vi "ARN Test Konfig v2.vi"() -> ()   [LabVIEW 2020, in "EPA 1065.lvlib" / "ARN Test 1065-305.lvlib"]
uses:
  ARN Test 1065-305.lvlib
  Visualisierungs Elemente/Zahlen-Ausgabefeld.ctl
  Allgemeine Einstellungen.ctl
  Seiten/System Einstellungen V2/Analysatoren.ctl
  T90 1065-308/Modus.ctl
  Seiten/System Einstellungen V2/Gasflasche Auswahl.ctl
  Seiten/System Einstellungen V2/Konfig Gasflasche.ctl
  T90 1065-308/Ergebnis.ctl
  Aktion FGV ARN Daten.ctl
  Seiten/FT-IR/FGV FT-IR Gasliste Aktionen.ctl
  Aktion FGV ARN Test.ctl
  Sprachverwaltung/FGV Aktion Tabelle zerlegen.ctl
  Aktion FGV Graphen Daten.ctl
  Seiten/System Einstellungen V2/Aktion FGV Gasbottledefinition.ctl
  PDF_Interface/PDF Interface Helper/PDFResultPictures.ctl
  Aktion FGV ARN Protokoll.ctl
  Messdaten/Aktionen FGV Messdaten.ctl
  Allgemeine VIs/Aktion Wertaenderung Gasliste.ctl
  Aktion FGV Protokoll.ctl
  Seiten/Gaszuordnung AO/FGV Gaszuordnung Grenzen&Einheit Aktion.ctl
  Allgemeine VIs/Aktion Test Status.ctl
  Funktionstasten/Funktionstasten-Aktion.ctl
  Funktionstasten/Zustaende.ctl
  Seiten/FT-IR/FGV FT-IR Parameter.vi
  Allgemein/allgemeine Sub-VIs.lvlib
  Seiten/FT-IR/FT-IR.lvlib
  Messdaten/Messdaten.lvlib
  Seiten/Grafik/Grafik.lvlib
  Funktionstasten/Funktionstasten.lvlib
  Seiten/Gaszuordnung AO/Gaszuordnung AO.lvlib
  EPA 1065.lvlib
  Sprachverwaltung/Sprachverwaltung.lvlib
  Seiten/System Einstellungen V2/System Einstellungen V2.lvlib
  PDF_Interface/PDF Interface Helper/PDF Interface Helper.lvlib
  T90 1065-308/T90 Test 1065-308.lvlib
panel:
  out "ARN Result PDF":waveform(sgl)(graph) caption="T90"
  out "Ergebnis PDF FALSE":T1 caption="Ergebnis 2"
  out "Ergebnis PDF TRUE":T1 caption="Ergebnis 1"
  in  "Systemeinstellung":bool caption="Gasliste geändert"
  in  "Gasliste geändert":bool
  in  "Registerkarte":enum32{"Settings", "ARN Test", "Result"}(tab)
  in  "ARN Konfig Daten":T2={"Bearbeiter:"="", "Analysator"="FT-IR", "Komponente:"=0, "Gasflaschen Nr.:"="", "Accuracy"=0.0, "Sollwert"=0.0, "Modus"=0, "Pfad:"=path "D:/IAG_Data/Log", "Textname:"="", "CG Aufschaltzeit:"=120.0, "Einheit"="", "N2 Aufschaltzeit:"=120.0, "Gasflasche"=0, "Konfig Gasflasche"=FALSE} {"Gasflasche" items=["----"=10000, "IAG O2"=0, "IAG C2H2"=1, "IAG C2H4"=2, "IAG NH3 200"=3, "IAG NH3 2000"=4, "IAG NH3 3000"=5, "IAG CO 5%"=6, "IAG Propane 2%"=7, "IAG NO 1000"=8, "IAG SO2"=9, "IAG C3H6"=10, "IAG CO2"=11, "IAG CO"=12, "IAG N2O"=13, "IAG N2O 100"=14, "IAG NO2 1000"=15, "IAG NO2 100"=16, "IAG CH4"=17, "IAG Propane"=18, "IAG NO 5000"=19, "Hansi"=20, "IAG MG"=21]; "Komponente:" items=["N2O (300) LP 191C (1of2)"=3, "N2O (1000) LP 191C (2of2)"=29, "N2O autorange (1000)"=40]; "Modus" items=["CG zu PNS", "CG zu Entnahmestelle"]; "N2 Aufschaltzeit:" min=10.0; "CG Aufschaltzeit:" min=10.0}
  in  "Speichern":bool
  out "Einheit":string
  out "Komponente":string caption="Komponente:"
  out "Status":string
  out "ARN":waveform(sgl)(graph) caption="T90"
  in  "Test Start":bool
  in  "Abbrechen":bool
  out "Istwert":T7 caption="Istwert:" format="%.2f"
  out "Mwert":sgl format="%.3f"
  out "PMwert":sgl format="%.3f"
  in  "Textfile":bool caption="Abbrechen"
  out "Einheit Noise 2":string
  out "Einheit Wiederh. 2":string
  out "Einheit Genauigkeit 2":string
  out "Einheit Noise":string
  out "Einheit Wiederh.":string
  out "Ergebnis 3":T1
  out "Ergebnis 2":T1
  out "Ergebnis 1":T1
  out "Rauschen":string
  out "Rauschen Grenze":string caption="Rauschen:"
  out "Wiederholgenauigkeit":string
  out "Genauigkeit":string
  out "Wiederholgenauigkeit Grenze":string caption="Wiederholgenauigkeit:"
  out "Genauigkeit Grenze":string caption="Genauigkeit:"
  out "Einheit Genauigkeit":string
  out "ARN Result":waveform(sgl)(graph) caption="T90"
  in  "Print PDF":bool caption="Abbrechen"
  out "Tabelle":string[][](table)
  out "Komponente 2":string caption="Komponente:"
  # "ANR Test EPA §1065.305"
  # "Allgemeine Einstellungen"
  # "Protokoll Einstellung"
  # "%"
  # "sec."
  # "sec."
  # "±"
  # "x"
  # "Grenzen"
  # "Ergebnis"
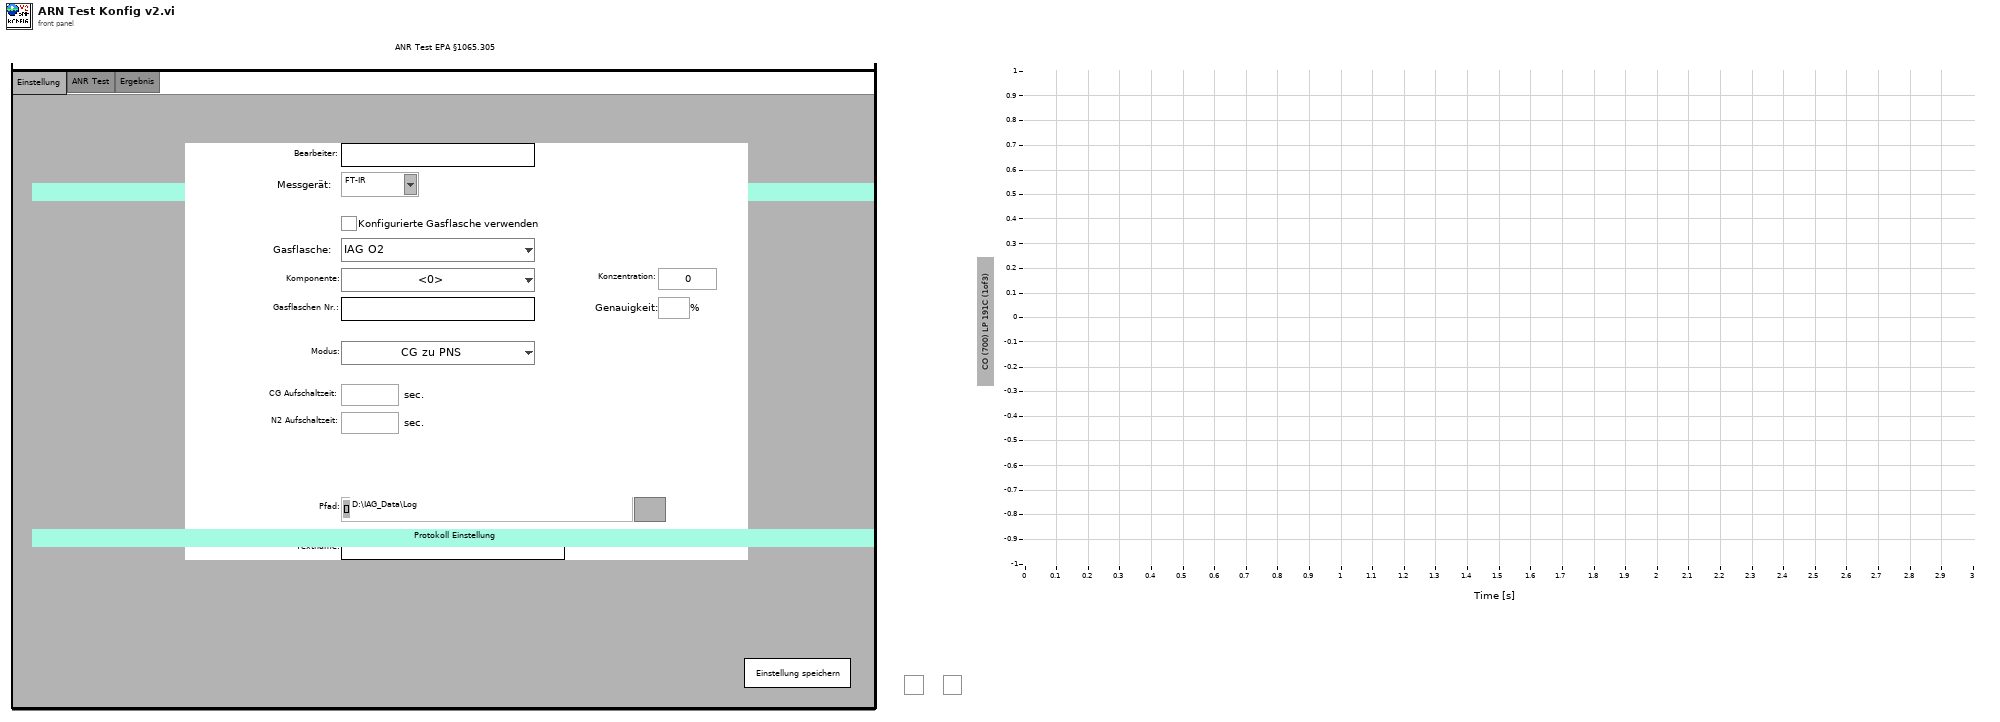
[diagram p1: front panel]
types:
  T1 = typedef "EPA 1065.lvlib/T90 Test 1065-308.lvlib/Ergebnis.ctl" = bool
  T2 = typedef "EPA 1065.lvlib/ARN Test 1065-305.lvlib/Allgemeine Einstellungen.ctl" = cluster{"Bearbeiter:":string, "Analysator":T3, "Komponente:":u16, "Gasflaschen Nr.:":string, "Accuracy":dbl, "Sollwert":dbl, "Modus":T4, "Pfad:":path, "Textname:":string, "CG Aufschaltzeit:":dbl, "Einheit":string, "N2 Aufschaltzeit:":dbl, "Gasflasche":T5, "Konfig Gasflasche":T6}
  T3 = typedef "System Einstellungen V2.lvlib/Analysatoren.ctl" = string
  T4 = typedef "EPA 1065.lvlib/T90 Test 1065-308.lvlib/Modus.ctl" = u16
  T5 = typedef "System Einstellungen V2.lvlib/Gasflasche Auswahl.ctl" = u16
  T6 = typedef "System Einstellungen V2.lvlib/Konfig Gasflasche.ctl" = bool
  T7 = typedef "Zahlen-Ausgabefeld.ctl" = sgl
  T8 = typedef "System Einstellungen V2.lvlib/Aktion FGV Gasbottledefinition.ctl" = enum16{"lesen", "schreiben", "löschen", "laden", "speichern", "exportieren", "importieren"}
  T9 = typedef "EPA 1065.lvlib/ARN Test 1065-305.lvlib/Aktion FGV ARN Daten.ctl" = enum16{"Lesen", "laden", "speichern", "ARN Daten", "Rohdaten", "Rohdaten löschen", "Zeitstempel", "SNR Ergebnis"}
  T10 = typedef "EPA 1065.lvlib/ARN Test 1065-305.lvlib/Aktion FGV Graphen Daten.ctl" = enum16{"init", "lesen", "Daten schreiben"}
  T11 = typedef "Sprachverwaltung.lvlib/FGV Aktion Tabelle zerlegen.ctl" = enum16{"laden", "vereinzeln", "speichern"}
  T12 = enum16{"init", "lesen", "ARN Test aktiv", "ARN Test inaktiv"}
  T13 = typedef "EPA 1065.lvlib/ARN Test 1065-305.lvlib/Aktion FGV ARN Test.ctl" = enum16{"leerlauf", "init", "lesen", "CG aufschalten", "Aufschaltzeit abwarten", "aufzeichnen vorbereiten", "aufzeichnen", "berechnen", "auswerten", "fertig", "0-Gas aufschalten", "0-Gas abwarten"}
  T14 = typedef "FT-IR.lvlib/FGV FT-IR Gasliste Aktionen.ctl" = enum16{"lesen", "Gasliste FT-IR", "Gasliste ausgelesen", "laden", "speichern", "löschen"}
  T15 = typedef "PDF Interface.lvlib/PDF Interface Helper.lvlib/PDFResultPictures.ctl" = cluster{"Yes Ctl Refnum":refnum<vi>, "No Ctl Refnum":refnum<vi>}
  T16 = typedef "String - Ausgabefeld.ctl" = string
  T17 = typedef "System Einstellungen V2.lvlib/Gasflasche gesamt.ctl" = cluster{"Gasflasche":T18, "Trägergas":T19, "Komponenten":T20[]}
  T18 = typedef "System Einstellungen V2.lvlib/Gasflasche.ctl" = cluster{"Gasname für die Auswahl":string, "Chargennummer":string, "Ablaufdatum":timestamp}
  T19 = typedef "System Einstellungen V2.lvlib/Traegergas.ctl" = string
  T20 = typedef "System Einstellungen V2.lvlib/Gasflaschenkomponente.ctl" = cluster{"Gasauswahl":string, "Konzentration IST":dbl, "Einheit":string, "Genauigkeit":dbl}
  T21 = cluster{"Komponente:":u16, "Sollwert":dbl, "Accuracy":dbl, "Einheit":string, "Gasflaschen Nr.:":string}
  T22 = typedef "EPA 1065.lvlib/Aktion Wertaenderung Gasliste.ctl" = enum16{"Init", "lesen", "Gasliste geändert", "ARN inaktiv", "LEAK inaktiv", "Interference 366 inaktiv", "T90 inaktiv", "Interference 375 inaktiv", "Chiller inaktiv", "FID O2 inaktiv", "FID Opti inaktiv", "Drift inaktiv", "Pre Test inaktiv", "LinV2 inaktiv", "HovaCAL Interference inaktiv"}
  T23 = typedef "Messdaten.lvlib/Aktionen FGV Messdaten.ctl" = enum16{"lesen", "schreiben", "löschen", "Mittelwerte", "Komponente"}
  T24 = typedef "EPA 1065.lvlib/ARN Test 1065-305.lvlib/Aktion FGV ARN Protokoll.ctl" = enum16{"lesen", "Tab. schreiben", "Protokoll ausw.", "Protokoll speichern", "Textdatei speichern"}
  T25 = typedef "EPA 1065.lvlib/ARN Test 1065-305.lvlib/Aktion FGV Protokoll.ctl" = enum16{"lesen", "schreiben", "Graph"}
  T26 = typedef "Gaszuordnung AO.lvlib/FGV Gaszuordnung Grenzen&Einheit Aktion.ctl" = enum16{"Lesen", "Schreiben Min", "Schreiben Max", "Laden", "Speichern"}
  T27 = typedef "EPA 1065.lvlib/Aktion Test Status.ctl" = enum16{"init", "lesen", "prüfen", "Interference 366", "Interference 375", "Chiller läuft", "Drift läuft", "Pre Test läuft", "FID Optimization läuft", "FID Interference läuft", "HovaCAL Interference", "LinV2"}
  T28 = typedef "Funktionstasten.lvlib/Zustaende.ctl" = enum16{"Standby", "Pause", "Eco", "Messen", "Kalibrieren", "Spülen Filter", "Spülen Leitung", "Umgebungsluft", "0-Gas", "Cal-Gas", "CG zu PNS", "-------------", "Init 1", "Init 2", "Init 3", "Init 4", "Messen vorbereiten", "Messen durchführen", "Exit"}
  T29 = typedef "Funktionstasten.lvlib/Funktionstasten-Aktion.ctl" = enum16{"Initialisieren", "Zustand setzen", "Taste gedrückt", "Fehler speichern", "Lesen", "Manuell", "Remote", "Bitparallel", "Samplepoint", "Zeit Prüfen", "reset Umschalten"}
  T30 = typedef "EPA 1065.lvlib/Aktive Tests Cluster.ctl" = cluster{"ANR läuft":bool, "T90 läuft":bool, "Leak läuft":bool, "Interference 366 läuft":bool, "Interference 375 läuft":bool, "Chiller läuft":bool, "FID Interference läuft":bool, "FID optimization läuft":bool, "Drift läuft":bool, "Pre-test läuft":bool, "HovaCAL Interference läuft":bool, "LinV2 läuft":bool}
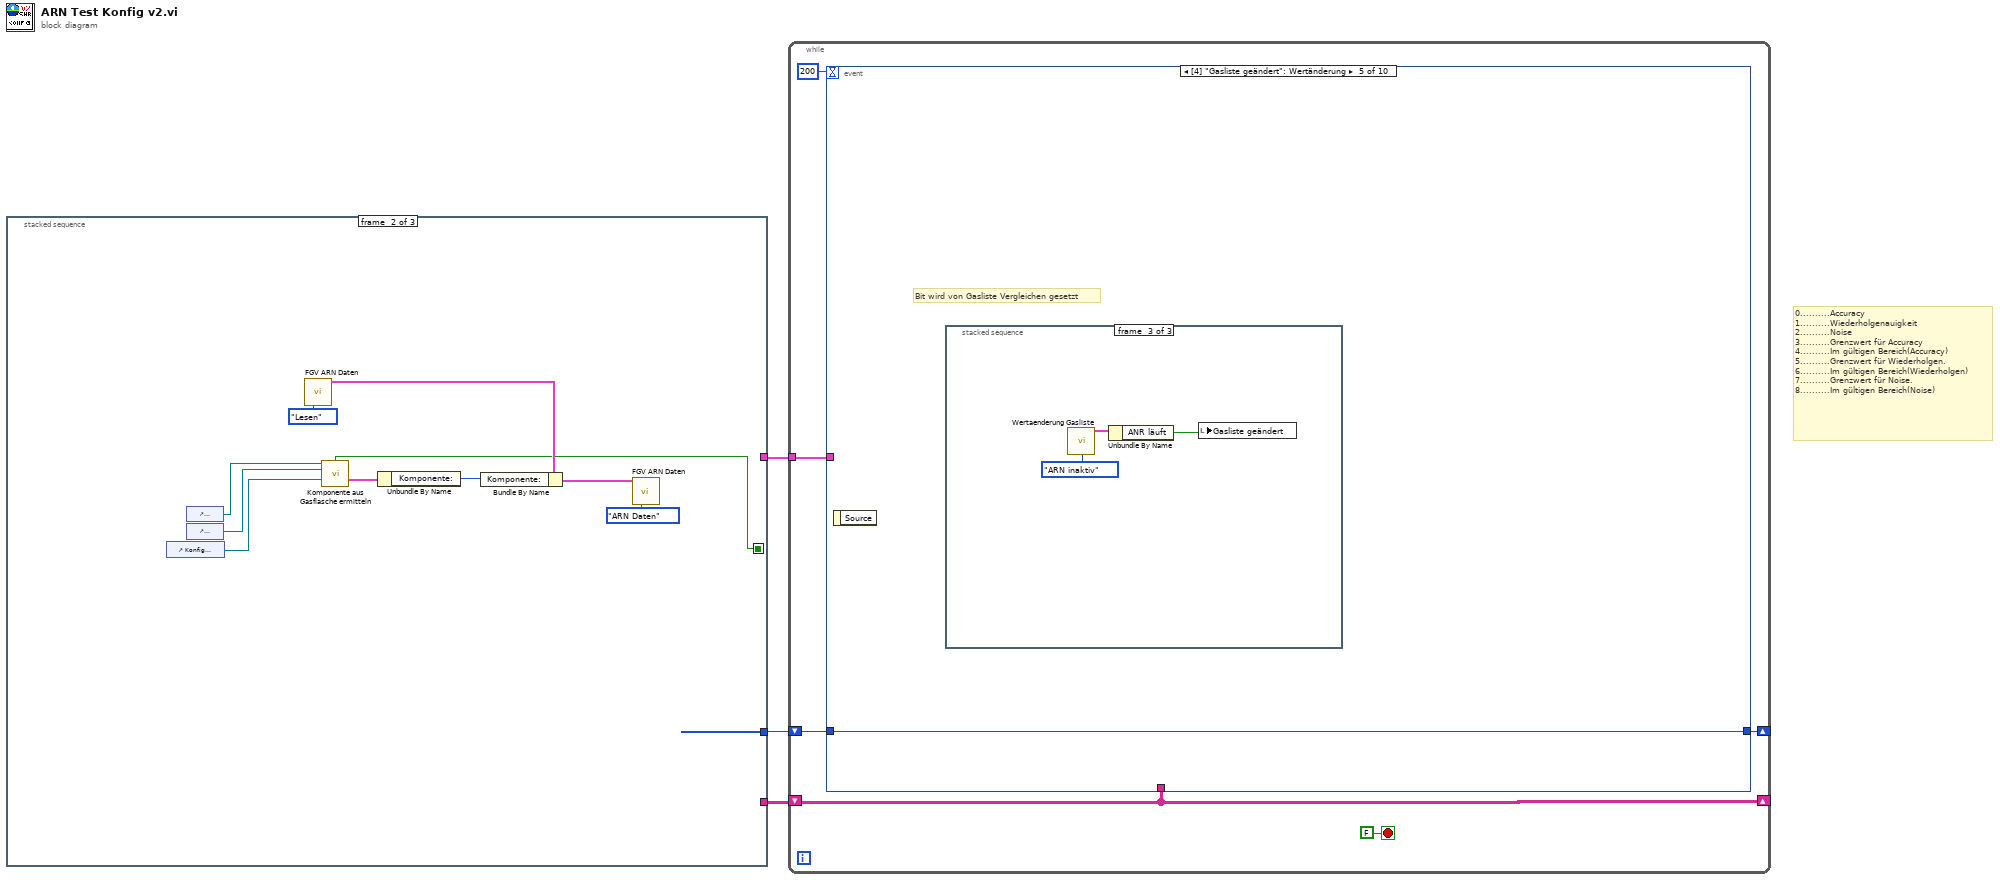
[diagram p0: block diagram]
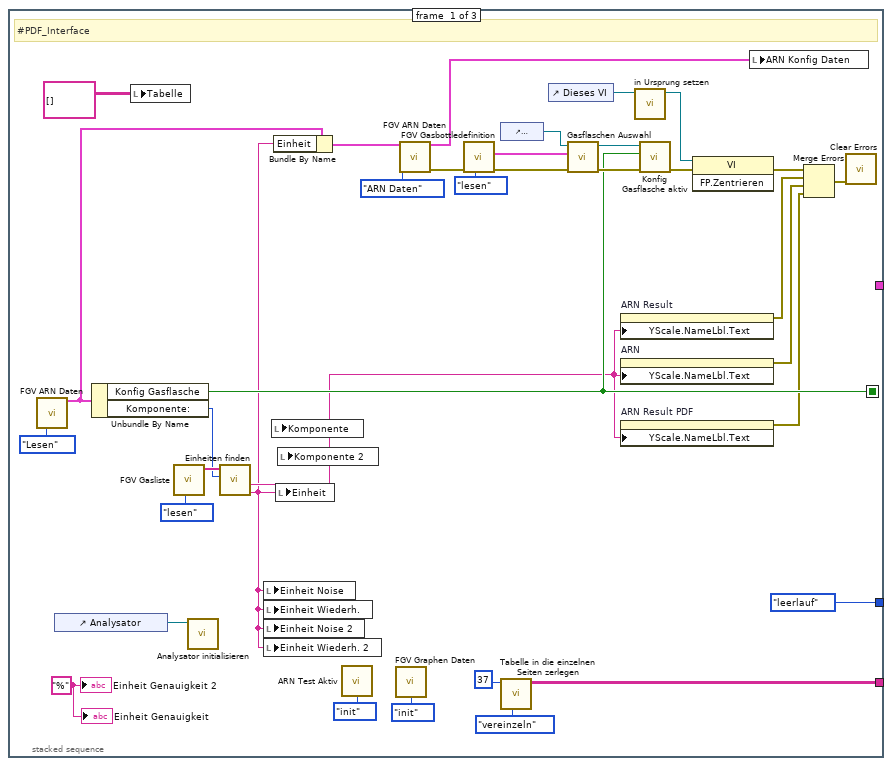
[diagram p2: hidden frame]
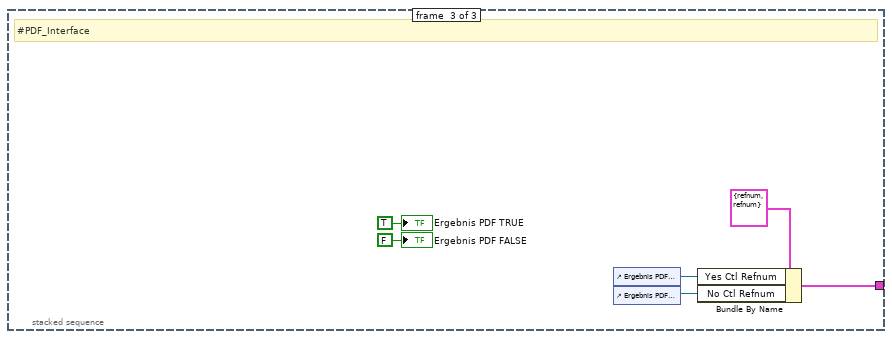
[diagram p3: hidden frame]
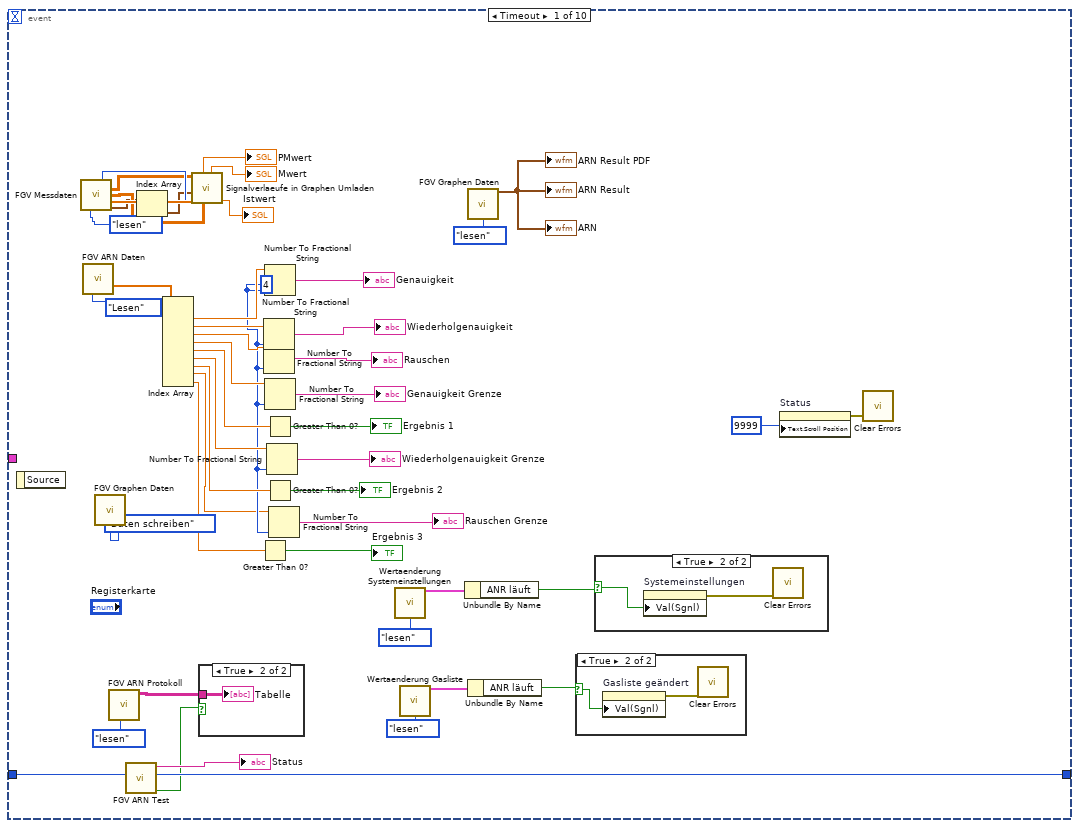
[diagram p4: hidden frame]
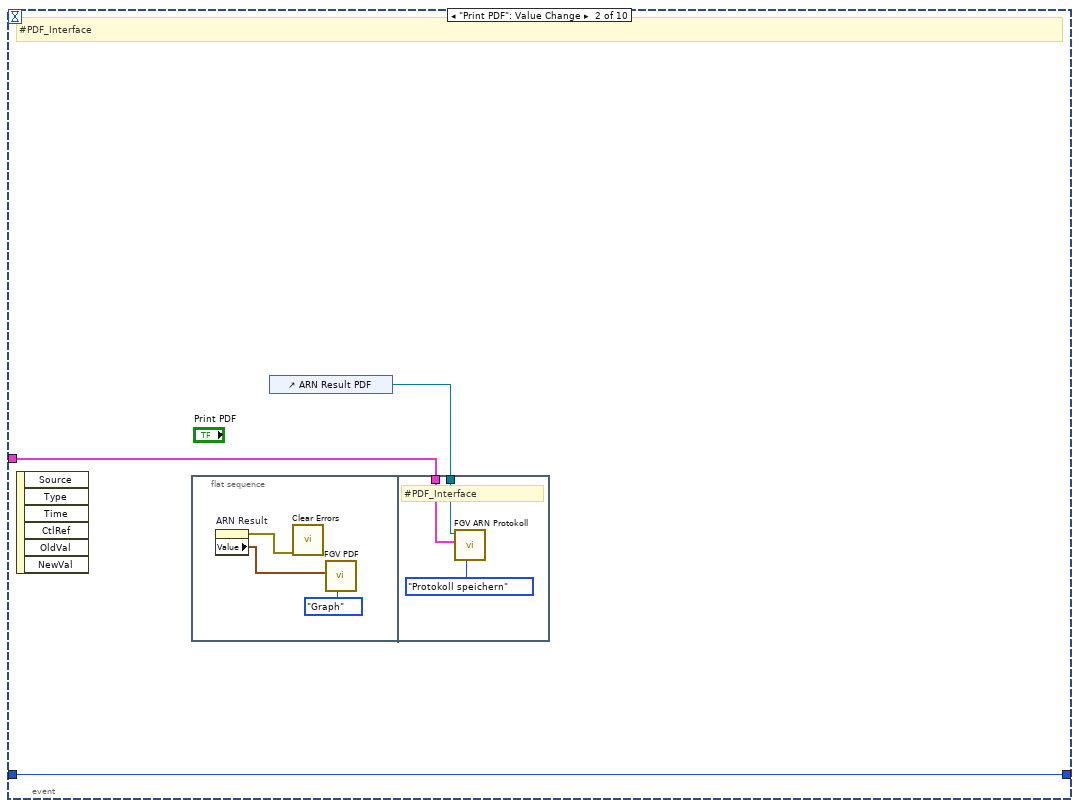
[diagram p8: hidden frame]
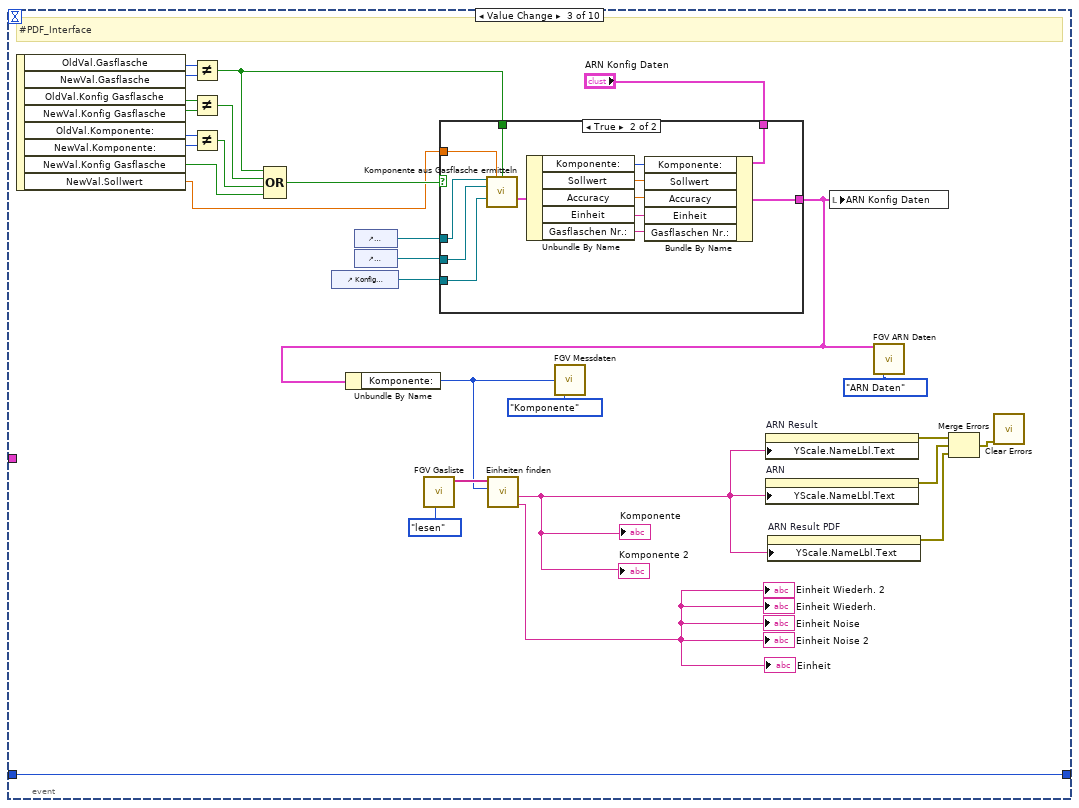
[diagram p9: hidden frame]
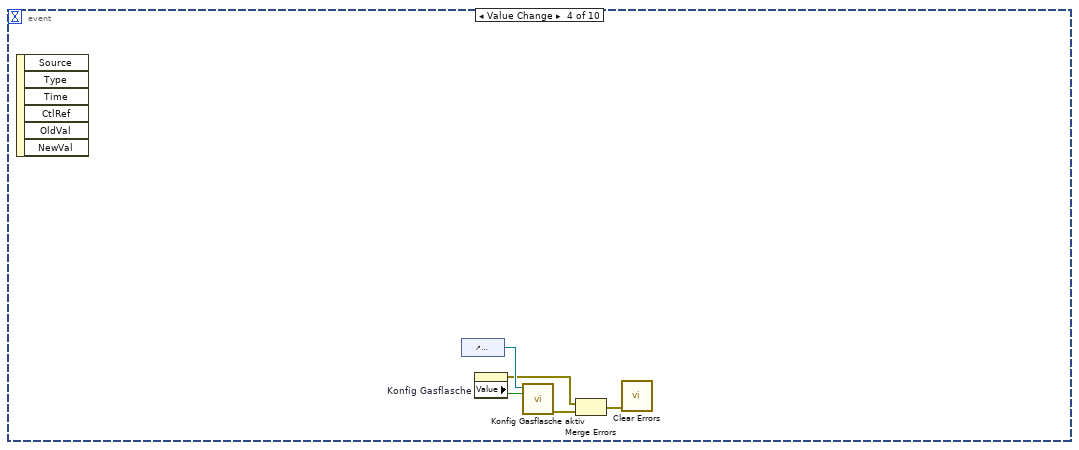
[diagram p11: hidden frame]
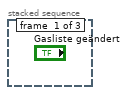
[diagram p12: hidden frame]
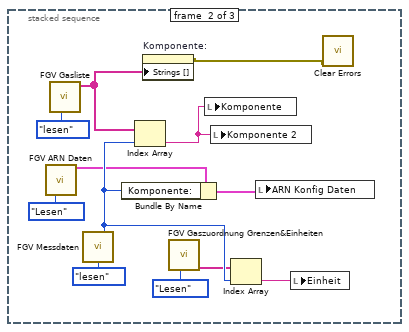
[diagram p13: hidden frame]
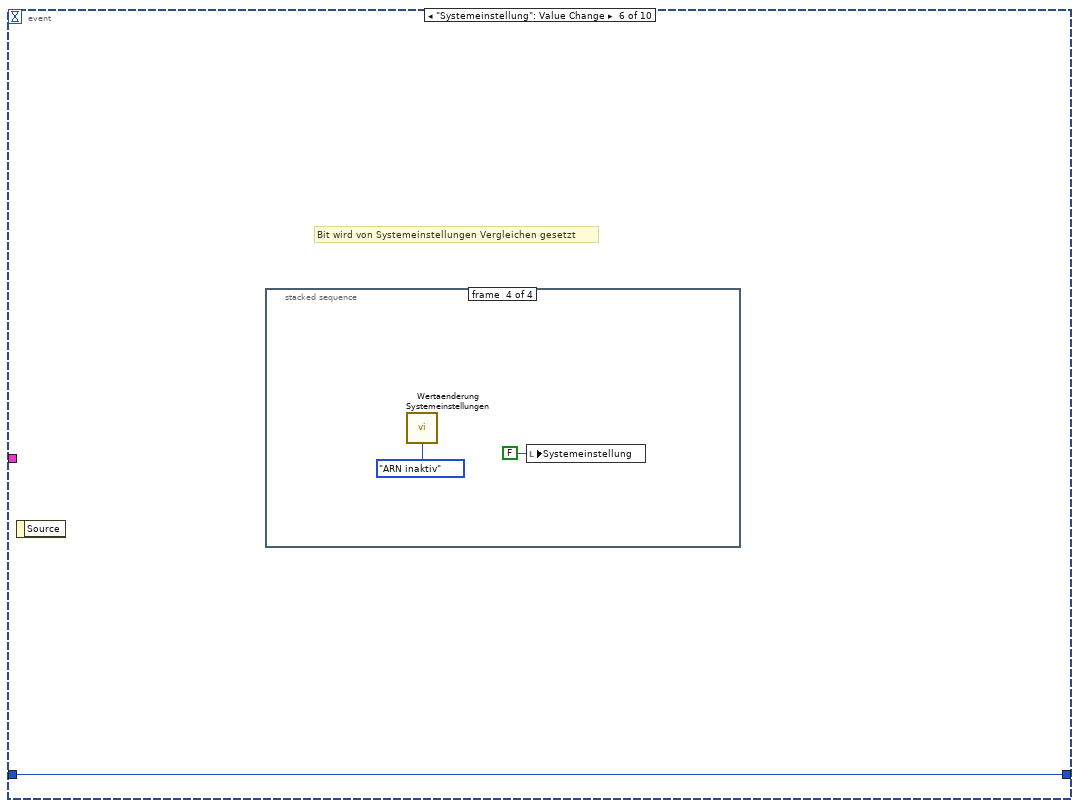
[diagram p14: hidden frame]
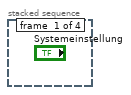
[diagram p15: hidden frame]
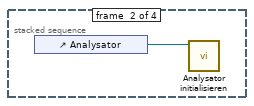
[diagram p16: hidden frame]
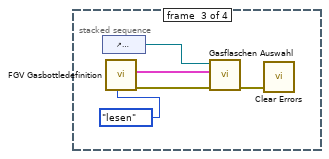
[diagram p17: hidden frame]
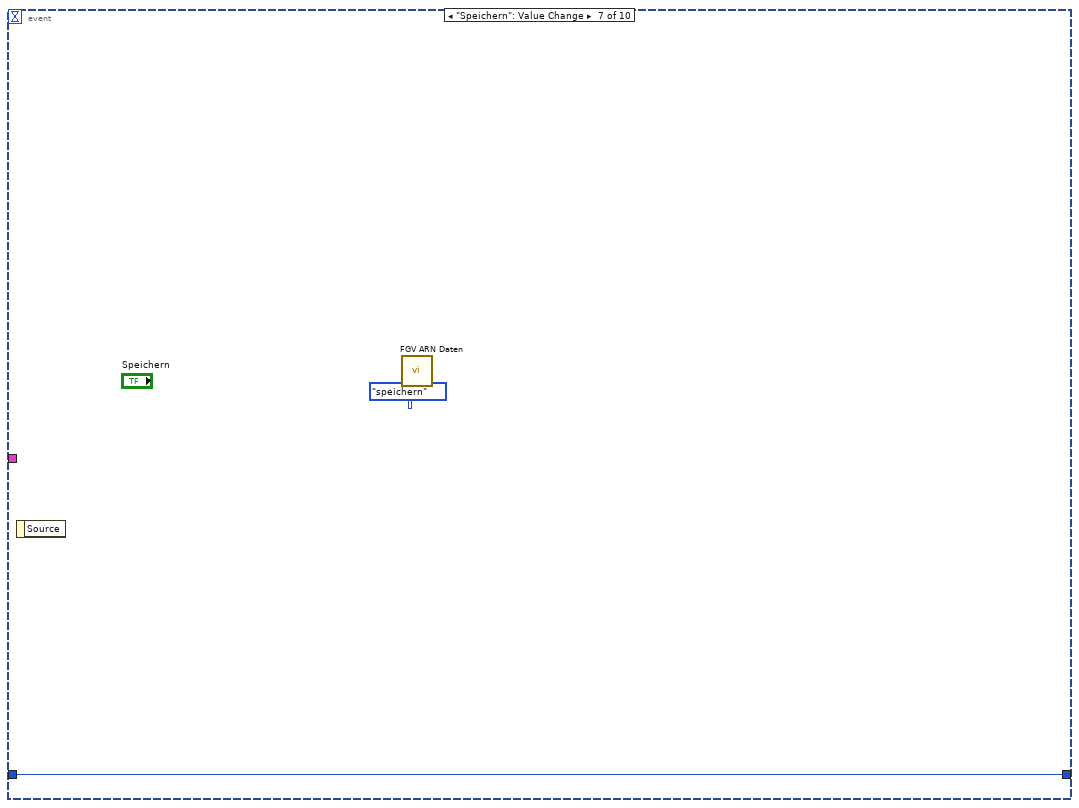
[diagram p18: hidden frame]
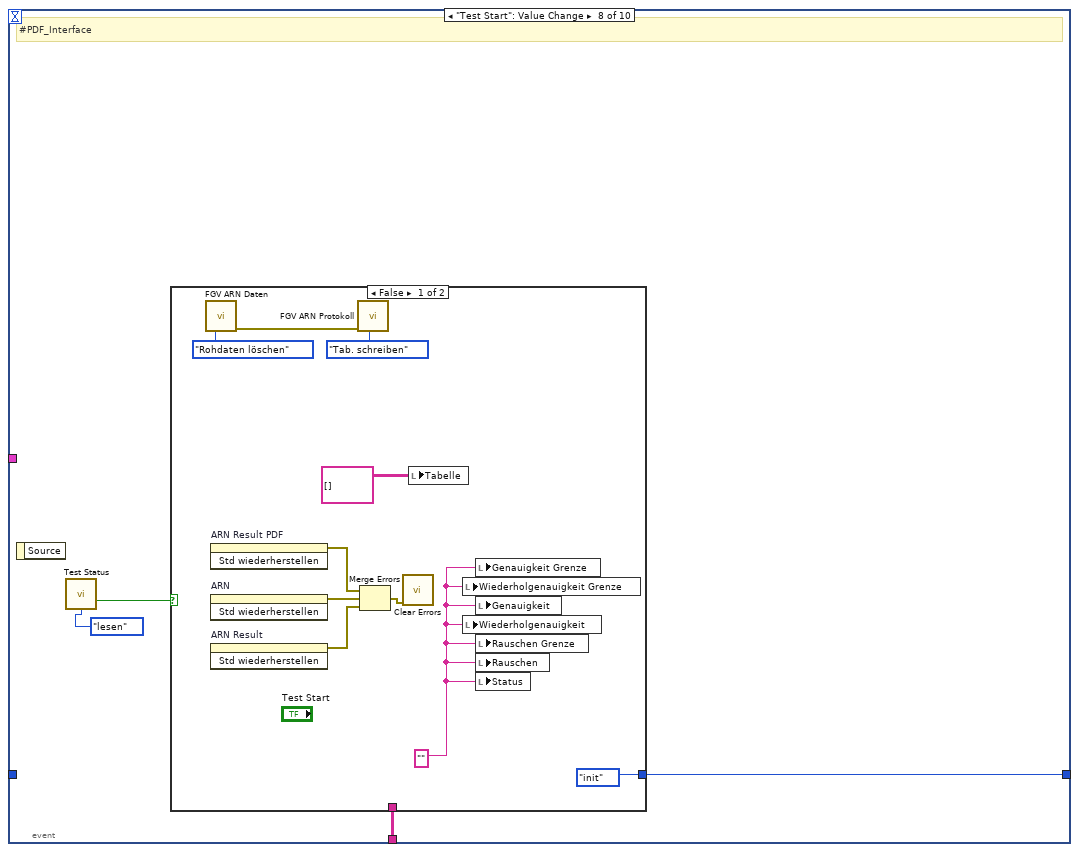
[diagram p19: hidden frame]
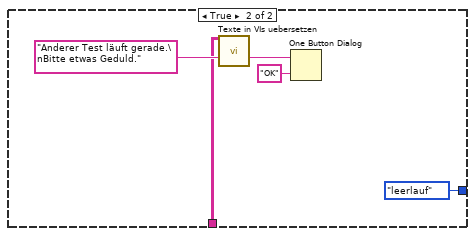
[diagram p20: hidden frame]
diagram:
  # "0..........Accuracy\n1..........Wiederholgenauigkeit\n2..........Noise\n3..........Grenzwert für Accuracy\n4..........Im gültigen Bereich(Accuracy)\n5..........Grenzwert für Wiederholgen.\n6..........Im gültigen Bereich(Wiederholgen)\n7..........Grenzwert für Noise.\n8..........Im gültigen Bereich(Noise)"
  n1 = stacked-sequence {
    seq-local: [w10 _ _] -> [_ w38 _]
    tunnel: [Aktion_FGV_ARN_Test."leerlauf" ("Aktion") _ _] -> w3
    tunnel: [w27 _ _] -> w2
    tunnel: [_ _ w48] -> w1
    frame #0 {
      w23 = "%" ("Einheit Genauigkeit 2")
      # "#PDF_Interface"
      n2 = call "FGV ARN Daten.vi"("Aktion"=Aktion_FGV_ARN_Daten."Lesen") -> ("ARN Konfig Daten"=w20:T2)  [unwired: 9 in, 5 out]
      n3 = control-ref of="Analysator"() -> (w11:refnum<vi>)
      n4 = Unbundle By Name(w20) -> ("Konfig Gasflasche"=w10:T6, "Komponente:"=w5:u16)
      n5 = local write "Tabelle"(string[][] [] ("Tabellenelement")) -> ()
      n6 = call "FGV Gasliste.vi"("Aktionen"=FGV_FT-IR_Gasliste_Aktionen."lesen") -> ("Aktuelle Gasliste FT-IR"=w8:T16[])  [unwired: 8 in, 2 out]
      n7 = call "Analysator initialisieren.vi"("Referenz Analysator"=w11) -> ()  [unwired: 9 in, 2 out]
      n8 = call "Einheiten finden.vi"("Komponente"=w5, "Aktuelle Gasliste gesamt"=w8) -> ("Einheit in String"=w6:string, "Komponenten Name"=w7:T16)  [unwired: 8 in]
      n9 = local write "Einheit Noise"(w6) -> ()
      n10 = local write "Einheit Wiederh."(w6) -> ()
      n11 = local write "Einheit Noise 2"(w6) -> ()
      n12 = local write "Einheit Wiederh. 2"(w6) -> ()
      n13 = local write "Komponente"(w7) -> ()
      n14 = Bundle By Name(cluster=w20, "Einheit"=w6) -> (w24:T2)
      n15 = local write "Einheit"(w6) -> ()
      n16 = local write "Komponente 2"(w7) -> ()
      n17 = call "ARN Test Aktiv.vi"("Aktion"=T12."init") -> ()  [unwired: 13 in, 2 out]
      n18 = call "FGV Graphen Daten.vi"("Aktion"=Aktion_FGV_Graphen_Daten."init") -> ()  [unwired: 12 in, 3 out]
      n19 = call "FGV ARN Daten.vi"("ARN Konfig Daten"=w24, "Aktion"=Aktion_FGV_ARN_Daten."ARN Daten") -> ("ARN Konfig Daten"=w14:T2, "error out"=w13:errorcluster)  [unwired: 8 in, 4 out]
      n20 = call "FGV Gasbottledefinition.vi"("Aktion"=Aktion_FGV_Gasbottledefinition."lesen", "error in (no error)"=w13) -> ("error out"=w19:errorcluster, "Gasflaschen Liste gesamt"=w18:T17[])  [unwired: 7 in, 1 out]
      n21 = control-ref of="Gasflasche"() -> (w17:refnum<vi>)
      n22 = call "Tabelle in die einzelnen Seiten zerlegen.vi"("Aktion"=FGV_Aktion_Tabelle_zerlegen."vereinzeln", "Index (Seite)"=37) -> ("Sprachliste"=w27:string[][])  [unwired: 7 in, 2 out]
      n23 = control-ref of="Dieses VI"() -> (w33:refnum<vi>)
      n24 = call "Gasflaschen Auswahl.vi"("error in (no error)"=w19, "Gasflaschen Liste gesamt"=w18, "Ring (Eingang)"=w17) -> ("error out"=w15:errorcluster)  [unwired: 8 in]
      n25 = property on="ARN Result" class="SVGraph (strikt)"("YScale.NameLbl.Text"=w7) -> (error out=w22:errorcluster)  [unwired: 2 in, 1 out]
      n26 = property on="ARN" class="SVGraph (strikt)"("YScale.NameLbl.Text"=w7) -> (error out=w21:errorcluster)  [unwired: 2 in, 1 out]
      n27 = property on="ARN Result PDF" class="SVGraph (strikt)"("YScale.NameLbl.Text"=w7) -> (error out=w9:errorcluster)  [unwired: 2 in, 1 out]
      n28 = call "in Ursprung setzen.vi"("VI Referenz"=w33) -> ("Referenz (Ausgang)"=w4:refnum<vi>)  [unwired: 10 in]
      n29 = call "Konfig Gasflasche aktiv.vi"("error in (no error)"=w15, "Konfig Gasflasche"=w10, "Referenz Gasflasche"=w17) -> ("error out"=w12:errorcluster)  [unwired: 8 in]
      n30 = invoke class="VI" method="FP.Zentrieren"(reference=w4, error in=w12) -> (error out=w32:errorcluster)  [unwired: 1 in, 2 out]
      n31 = local write "ARN Konfig Daten"(w14) -> ()
      n32 = Merge Errors(w32, w22, w21, w9) -> (w34:errorcluster)
      n33 = call <vilib>:"Clear Errors.vi"("error in (no error)"=w34) -> ()  [unwired: 5 in, 2 out]
      "Einheit Genauigkeit" <- w23
      "Einheit Genauigkeit 2" <- w23
    }
    frame #1 {
      n34 = control-ref of="Konfig Gasflasche"() -> (w43:refnum<vi>)
      n35 = control-ref of="Gasflasche"() -> (w45:refnum<vi>)
      n36 = control-ref of="Komponente:"() -> (w44:refnum<vi>)
      n37 = call "FGV ARN Daten.vi"("Aktion"=Aktion_FGV_ARN_Daten."Lesen") -> ("ARN Konfig Daten"=w42:T2)  [unwired: 9 in, 5 out]
      n38 = call "Komponente aus Gasflasche ermitteln.vi"("Referenz Gasflasche"=w45, "Wertänderung Gasflasche"=w38, "Referenz Komponente"=w44, "Referenz Konfig Gasflasche"=w43) -> ("Ausgangs-Cluster"=w41:T21)  [unwired: 8 in, 3 out]
      n39 = Unbundle By Name(w41) -> ("Komponente:"=w40:u16)
      n40 = Bundle By Name(cluster=w42, "Komponente:"=w40) -> (w39:T2)
      n41 = call "FGV ARN Daten.vi"("ARN Konfig Daten"=w39, "Aktion"=Aktion_FGV_ARN_Daten."ARN Daten") -> ()  [unwired: 8 in, 6 out]
    }
    frame #2 {
      # "#PDF_Interface"
      n42 = control-ref of="Ergebnis PDF TRUE"() -> (w51:refnum<vi>)
      n43 = control-ref of="Ergebnis PDF FALSE"() -> (w50:refnum<vi>)
      n44 = Bundle By Name(cluster=T15 {"Yes Ctl Refnum"=refnum, "No Ctl Refnum"=refnum} ("ResultPictures"), "Yes Ctl Refnum"=w51, "No Ctl Refnum"=w50) -> (w48:T15)
      "Ergebnis PDF TRUE" <- T1 TRUE ("Ergebnis PDF TRUE")
      "Ergebnis PDF FALSE" <- T1 FALSE ("Ergebnis PDF FALSE")
    }
  }
  n45 = while {
    shift-right: [w56] -> _
    shift-left: w3 -> [w57]
    shift-right: [w55] -> _
    shift-left: w2 -> [w55]
    tunnel: w1 -> [w54]
    stop <- FALSE stop-if-true
    n46 = event shown="[4] \"Gasliste geändert\": Wertänderung" {
      selector: _ -> [_ _ _ _ _ _ _ _ _ _]
      dyn-events: _ -> [_ _ _ _ _ _ _ _ _ _]
      timeout: 200 -> [_ _ _ _ _ _ _ _ _ _]
      tunnel: w57 -> [w95 w115 w150 _ w170 w186 w196 _ w216 w230]
      tunnel: [w94 w115 w150 _ w170 w186 w196 w200 w222 w230] -> w56
      tunnel: w55 -> [_ _ _ _ _ _ _ w197 _ _]
      tunnel: w54 -> [_ w114 _ _ _ _ _ _ _ _]
      event Timeout {
        w75 = i16 4 ("Genauigkeit (6)")
        n47 = event-data() -> ()  [unwired: 1 in, 1 out]
        n48 = call "FGV Messdaten.vi"("Aktionen"=Aktionen_FGV_Messdaten."lesen") -> ("Komponente"=w102:u16, "Messdaten"=w99:sgl[][], "Mittelwertdaten"=w103:sgl[][], "Deviation"=w104:sgl[], "Zeitstempeln"=w97:timestamp[])  [unwired: 6 in, 4 out]
        n49 = call "FGV ARN Daten.vi"("Aktion"=Aktion_FGV_ARN_Daten."Lesen") -> ("SNR Ergebnis"=w105:sgl[])  [unwired: 9 in, 5 out]
        n50 = call "FGV Graphen Daten.vi"("Aktion"=Aktion_FGV_Graphen_Daten."Daten schreiben") -> ()  [unwired: 12 in, 3 out]
        n51 = call "FGV ARN Protokoll.vi"("Aktion"=Aktion_FGV_ARN_Protokoll."lesen") -> ("Tabelle"=w70:string[][])  [unwired: 8 in, 2 out]
        n52 = call "FGV ARN Test.vi"("Aktion"=w95) -> ("Tabelle Wertänderung"=w68:bool, "Aktion"=w94:T13, "Status"=→"Status":string)  [unwired: 7 in, 1 out]
        n53 = Index Array(array=w97) -> (element=w98:timestamp)  [unwired: 1 in]
        n54 = Index Array(array=w105) -> (element #1=w89:sgl, element #2=w87:sgl, element #3=w85:sgl, element #4=w83:sgl, element #5=w81:sgl, element #6=w79:sgl, element #7=w77:sgl, element #8=w74:sgl, element #9=w72:sgl)  [unwired: 9 in]
        n55 = call "Signalverlaeufe in Graphen Umladen.vi"("Deviation"=w104, "Mittelwertdaten"=w103, "Gas-Auswahl"=w102, "t0"=w98, "Werte"=w99) -> ("Konzentration"=→"Istwert":sgl, "aktuelle Mittelwert"=→"Mwert":sgl, "Deviation"=→"PMwert":sgl)  [unwired: 2 in, 2 out]
        n56 = case shown="True" w68 {
          tunnel: w70 -> [_ w112]
          frame False {
          }
          frame True {
            "Tabelle" <- w112
          }
        }
        n57 = Greater Than 0?(x=w72) -> (x > 0?=→"Ergebnis 3":bool)
        n58 = Number To Fractional String(number=w87, precision (6)=w75) -> (F-format string=→"Wiederholgenauigkeit":string)  [unwired: 2 in]
        n59 = Number To Fractional String(number=w85, precision (6)=w75) -> (F-format string=→"Rauschen":string)  [unwired: 2 in]
        n60 = Number To Fractional String(number=w89, precision (6)=w75) -> (F-format string=→"Genauigkeit":string)  [unwired: 2 in]
        n61 = Number To Fractional String(number=w83, precision (6)=w75) -> (F-format string=→"Genauigkeit Grenze":string)  [unwired: 2 in]
        n62 = Greater Than 0?(x=w81) -> (x > 0?=→"Ergebnis 1":bool)
        n63 = Greater Than 0?(x=w77) -> (x > 0?=→"Ergebnis 2":bool)
        n64 = Number To Fractional String(number=w79, precision (6)=w75) -> (F-format string=→"Wiederholgenauigkeit Grenze":string)  [unwired: 2 in]
        n65 = Number To Fractional String(number=w74, precision (6)=w75) -> (F-format string=→"Rauschen Grenze":string)  [unwired: 2 in]
        n66 = call "Wertaenderung Systemeinstellungen.vi"("Aktion"=Aktion_Wertaenderung_Gasliste."lesen") -> ("Tests"=w62:T30)  [unwired: 13 in, 1 out]
        n67 = call "Wertaenderung Gasliste.vi"("Aktion"=Aktion_Wertaenderung_Gasliste."lesen") -> ("Tests"=w65:T30)  [unwired: 13 in, 1 out]
        n68 = Unbundle By Name(w62) -> ("ANR läuft"=w61:bool)
        n69 = call "FGV Graphen Daten.vi"("Aktion"=Aktion_FGV_Graphen_Daten."lesen") -> ("Waveform"=→"ARN Result" →"ARN" →"ARN Result PDF":waveform(sgl))  [unwired: 12 in, 2 out]
        n70 = Unbundle By Name(w65) -> ("ANR läuft"=w64:bool)
        n71 = case shown="True" w64 {
          selector: w64 -> [_ w110]
          frame False {
          }
          frame True {
            n72 = property on="Gasliste geändert" class="Bool. (strikt)"("Val(Sgnl)"=w110) -> (error out=w111:errorcluster)  [unwired: 2 in, 1 out]
            n73 = call <vilib>:"Clear Errors.vi"("error in (no error)"=w111) -> ()  [unwired: 5 in, 2 out]
          }
        }
        n74 = case shown="True" w61 {
          selector: w61 -> [_ w108]
          frame False {
          }
          frame True {
            n75 = property on="Systemeinstellungen" class="Bool. (strikt)"("Val(Sgnl)"=w108) -> (error out=w109:errorcluster)  [unwired: 2 in, 1 out]
            n76 = call <vilib>:"Clear Errors.vi"("error in (no error)"=w109) -> ()  [unwired: 5 in, 2 out]
          }
        }
        n77 = property on="Status" class="Str"("Text.Scroll Position"=u32 9999 ("Text.Anzeigeposition")) -> (error out=w92:errorcluster)  [unwired: 2 in, 1 out]
        n78 = call <vilib>:"Clear Errors.vi"("error in (no error)"=w92) -> ()  [unwired: 5 in, 2 out]
      }
      event "Print PDF": Value Change {
        # "#PDF_Interface"
        n79 = event-data() -> ()  [unwired: 1 in, 6 out]
        n80 = flat-sequence {
          tunnel: w114 -> [w120]
          tunnel: w113 -> [w119]
          frame #0 {
            n81 = property on="ARN Result" class="SVGraph (strikt)"() -> (error out=w116:errorcluster, "Value"=w117:waveform(sgl))  [unwired: 2 in, 1 out]
            n82 = call <vilib>:"Clear Errors.vi"("error in (no error)"=w116) -> ()  [unwired: 5 in, 2 out]
            n83 = call "FGV PDF.vi"("Aktion"=Aktion_FGV_Protokoll."Graph", "Graph"=w117) -> ()  [unwired: 8 in, 2 out]
          }
          frame #1 {
            # "#PDF_Interface"
            n84 = call "FGV ARN Protokoll.vi"("Aktion"=Aktion_FGV_ARN_Protokoll."Protokoll speichern", "ResultPictures"=w120, "SVGraph Referenz"=w119) -> ()  [unwired: 6 in, 3 out]
          }
        }
        n85 = control-ref of="ARN Result PDF"() -> (w113:refnum<vi>)
      }
      event Value Change {
        # "#PDF_Interface"
        n86 = event-data() -> ("OldVal.Gasflasche"=w145:T5, "NewVal.Gasflasche"=w144:T5, "OldVal.Konfig Gasflasche"=w140:T6, "NewVal.Konfig Gasflasche"=w139:T6, "OldVal.Komponente:"=w138:u16, "NewVal.Komponente:"=w124:u16, "NewVal.Konfig Gasflasche"=w125:T6, "NewVal.Sollwert"=w122:dbl)  [unwired: 1 in]
        n87 = Not Equal?(x=w145, y=w144) -> (x != y?=w137:bool)
        n88 = Not Equal?(x=w140, y=w139) -> (x != y?=w136:T6)
        n89 = Not Equal?(x=w138, y=w124) -> (x != y?=w135:bool)
        n90 = Compound Arithmetic op=OR ("Mehrfacharithmetik")(w137, w136, w135, w125) -> (w134:T6)
        n91 = control-ref of="Konfig Gasflasche"() -> (w133:refnum<vi>)
        n92 = control-ref of="Gasflasche"() -> (w131:refnum<vi>)
        n93 = control-ref of="Komponente:"() -> (w132:refnum<vi>)
        n94 = call "FGV Gasliste.vi"("Aktionen"=FGV_FT-IR_Gasliste_Aktionen."lesen") -> ("Aktuelle Gasliste FT-IR"=w129:T16[])  [unwired: 8 in, 2 out]
        n95 = case shown="True" w134 {
          tunnel: w137 -> [_ w164]
          tunnel: "ARN Konfig Daten" -> [w151 w161]
          tunnel: [w151 w160] -> w126
          tunnel: w133 -> [_ w159]
          tunnel: w132 -> [_ w157]
          tunnel: w131 -> [_ w158]
          tunnel: w122 -> [_ w152]
          frame False {
          }
          frame True {
            n96 = call "Komponente aus Gasflasche ermitteln.vi"("Referenz Gasflasche"=w158, "Konzentration IST"=w152, "Wertänderung Gasflasche"=w164, "Referenz Komponente"=w157, "Referenz Konfig Gasflasche"=w159) -> ("Ausgangs-Cluster"=w162:T21)  [unwired: 7 in, 3 out]
            n97 = Unbundle By Name(w162) -> ("Komponente:"=w156:u16, "Sollwert"=w155:dbl, "Accuracy"=w154:dbl, "Einheit"=w163:string, "Gasflaschen Nr.:"=w153:string)
            n98 = Bundle By Name(cluster=w161, "Komponente:"=w156, "Sollwert"=w155, "Accuracy"=w154, "Einheit"=w163, "Gasflaschen Nr.:"=w153) -> (w160:T2)
          }
        }
        n99 = Unbundle By Name(w126) -> ("Komponente:"=w128:u16)
        n100 = call "Einheiten finden.vi"("Komponente"=w128, "Aktuelle Gasliste gesamt"=w129) -> ("Einheit in String"=→"Einheit" →"Einheit Wiederh. 2" →"Einheit Noise 2" →"Einheit Wiederh." →"Einheit Noise":string, "Komponenten Name"=w127:T16)  [unwired: 8 in]
        "Komponente" <- w127
        "Komponente 2" <- w127
        n101 = call "FGV Messdaten.vi"("Komponente"=w128, "Aktionen"=Aktionen_FGV_Messdaten."Komponente") -> ()  [unwired: 5 in, 9 out]
        n102 = property on="ARN Result" class="SVGraph (strikt)"("YScale.NameLbl.Text"=w127) -> (error out=w147:errorcluster)  [unwired: 2 in, 1 out]
        n103 = property on="ARN" class="SVGraph (strikt)"("YScale.NameLbl.Text"=w127) -> (error out=w148:errorcluster)  [unwired: 2 in, 1 out]
        n104 = property on="ARN Result PDF" class="SVGraph (strikt)"("YScale.NameLbl.Text"=w127) -> (error out=w130:errorcluster)  [unwired: 2 in, 1 out]
        n105 = local write "ARN Konfig Daten"(w126) -> ()
        n106 = call "FGV ARN Daten.vi"("ARN Konfig Daten"=w126, "Aktion"=Aktion_FGV_ARN_Daten."ARN Daten") -> ()  [unwired: 8 in, 6 out]
        n107 = Merge Errors(w147, w148, w130) -> (w149:errorcluster)
        n108 = call <vilib>:"Clear Errors.vi"("error in (no error)"=w149) -> ()  [unwired: 5 in, 2 out]
      }
      event Value Change {
        n109 = event-data() -> ()  [unwired: 1 in, 6 out]
        n110 = control-ref of="Gasflasche"() -> (w168:refnum<vi>)
        n111 = property on="Konfig Gasflasche" class="Bool. (strikt)"() -> (error out=w166:errorcluster, "Value"=w169:T6)  [unwired: 2 in, 1 out]
        n112 = call "Konfig Gasflasche aktiv.vi"("Konfig Gasflasche"=w169, "Referenz Gasflasche"=w168) -> ("error out"=w165:errorcluster)  [unwired: 9 in]
        n113 = Merge Errors(w166, w165) -> (w167:errorcluster)
        n114 = call <vilib>:"Clear Errors.vi"("error in (no error)"=w167) -> ()  [unwired: 5 in, 2 out]
      }
      event "Gasliste geändert": Value Change {
        # "Bit wird von Gasliste Vergleichen gesetzt"
        n115 = event-data() -> ()  [unwired: 1 in, 1 out]
        n116 = stacked-sequence {
          frame #0 {
          }
          frame #1 {
            n117 = call "FGV ARN Daten.vi"("Aktion"=Aktion_FGV_ARN_Daten."Lesen") -> ("ARN Konfig Daten"=w176:T2)  [unwired: 9 in, 5 out]
            n118 = call "FGV Gasliste.vi"("Aktionen"=FGV_FT-IR_Gasliste_Aktionen."lesen") -> ("Aktuelle Gasliste FT-IR"=w171:T16[])  [unwired: 8 in, 2 out]
            n119 = call "FGV Messdaten.vi"("Aktionen"=Aktionen_FGV_Messdaten."lesen") -> ("Komponente"=w180:u16)  [unwired: 6 in, 8 out]
            n120 = Bundle By Name(cluster=w176, "Komponente:"=w180) -> (w177:T2)
            n121 = Index Array(array=w171, index=w180) -> (element=w182:T16)
            n122 = property on="Komponente:" class="Ring (strikt)"("Strings []"=w171) -> (error out=w172:errorcluster)  [unwired: 2 in, 1 out]
            n123 = call "FGV Gaszuordnung Grenzen&Einheiten.vi"("Aktion"=FGV_Gaszuordnung_Grenzen&Einheit_Aktion."Lesen") -> ("Einheit neu"=w179:string[])  [unwired: 2 in, 8 out]
            n124 = local write "Komponente"(w182) -> ()
            n125 = local write "Komponente 2"(w182) -> ()
            n126 = Index Array(array=w179, index=w180) -> (element=w181:string)
            n127 = local write "ARN Konfig Daten"(w177) -> ()
            n128 = local write "Einheit"(w181) -> ()
            n129 = call <vilib>:"Clear Errors.vi"("error in (no error)"=w172) -> ()  [unwired: 5 in, 2 out]
          }
          frame #2 {
            n130 = call "Wertaenderung Gasliste.vi"("Aktion"=Aktion_Wertaenderung_Gasliste."ARN inaktiv") -> ("Tests"=w184:T30)  [unwired: 13 in, 1 out]
            n131 = Unbundle By Name(w184) -> ("ANR läuft"=w183:bool)
            n132 = local write "Gasliste geändert"(w183) -> ()
          }
        }
      }
      event "Systemeinstellung": Value Change {
        # "Bit wird von Systemeinstellungen Vergleichen gesetzt"
        n133 = event-data() -> ()  [unwired: 1 in, 1 out]
        n134 = stacked-sequence {
          frame #0 {
          }
          frame #1 {
            n135 = control-ref of="Analysator"() -> (w187:refnum<vi>)
            n136 = call "Analysator initialisieren.vi"("Referenz Analysator"=w187) -> ()  [unwired: 9 in, 2 out]
          }
          frame #2 {
            n137 = control-ref of="Gasflasche"() -> (w190:refnum<vi>)
            n138 = call "FGV Gasbottledefinition.vi"("Aktion"=Aktion_FGV_Gasbottledefinition."lesen") -> ("error out"=w192:errorcluster, "Gasflaschen Liste gesamt"=w189:T17[])  [unwired: 8 in, 1 out]
            n139 = call "Gasflaschen Auswahl.vi"("error in (no error)"=w192, "Gasflaschen Liste gesamt"=w189, "Ring (Eingang)"=w190) -> ("error out"=w191:errorcluster)  [unwired: 8 in]
            n140 = call <vilib>:"Clear Errors.vi"("error in (no error)"=w191) -> ()  [unwired: 5 in, 2 out]
          }
          frame #3 {
            n141 = call "Wertaenderung Systemeinstellungen.vi"("Aktion"=Aktion_Wertaenderung_Gasliste."ARN inaktiv") -> ()  [unwired: 13 in, 2 out]
            n142 = local write "Systemeinstellung"(FALSE ("Systemeinstellung")) -> ()
          }
        }
      }
      event "Speichern": Value Change {
        n143 = event-data() -> ()  [unwired: 1 in, 1 out]
        n144 = call "FGV ARN Daten.vi"("Aktion"=Aktion_FGV_ARN_Daten."speichern") -> ()  [unwired: 9 in, 6 out]
      }
      event "Test Start": Value Change {
        # "#PDF_Interface"
        n145 = event-data() -> ()  [unwired: 1 in, 1 out]
        n146 = call "Test Status.vi"("Aktion"=Aktion_Test_Status."lesen") -> ("Tests sperren"=w198:bool)  [unwired: 11 in, 3 out]
        n147 = case shown="False" w198 {
          tunnel: [Aktion_FGV_ARN_Test."init" ("Aktion") Aktion_FGV_ARN_Test."leerlauf" ("Aktion")] -> w200
          tunnel: w197 -> [_ w211]
          frame False {
            w203 = "" ("Status")
            n148 = call "FGV ARN Daten.vi"("Aktion"=Aktion_FGV_ARN_Daten."Rohdaten löschen") -> ("error out"=w208:errorcluster)  [unwired: 9 in, 5 out]
            n149 = invoke on="ARN Result PDF" class="SVGraph (strikt)" method="Std wiederherstellen"() -> (error out=w201:errorcluster)  [unwired: 3 in, 2 out]
            n150 = invoke on="ARN" class="SVGraph (strikt)" method="Std wiederherstellen"() -> (error out=w205:errorcluster)  [unwired: 3 in, 2 out]
            n151 = invoke on="ARN Result" class="SVGraph (strikt)" method="Std wiederherstellen"() -> (error out=w204:errorcluster)  [unwired: 3 in, 2 out]
            n152 = call "FGV ARN Protokoll.vi"("Aktion"=Aktion_FGV_ARN_Protokoll."Tab. schreiben", "error in (no error)"=w208) -> ()  [unwired: 7 in, 3 out]
            n153 = Merge Errors(w201, w205, w204) -> (w206:errorcluster)
            n154 = call <vilib>:"Clear Errors.vi"("error in (no error)"=w206) -> ()  [unwired: 5 in, 2 out]
            n155 = local write "Tabelle"(string[][] [] ("Tabellenelement")) -> ()
            n156 = local write "Wiederholgenauigkeit Grenze"(w203) -> ()
            n157 = local write "Wiederholgenauigkeit"(w203) -> ()
            n158 = local write "Genauigkeit Grenze"(w203) -> ()
            n159 = local write "Genauigkeit"(w203) -> ()
            n160 = local write "Rauschen Grenze"(w203) -> ()
            n161 = local write "Rauschen"(w203) -> ()
            n162 = local write "Status"(w203) -> ()
          }
          frame True {
            n163 = call "Texte in VIs uebersetzen.vi"("Sprachliste"=w211, "String zum Übersetzen"="Anderer Test läuft gerade.\nBitte etwas Geduld." ("Nachricht")) -> ("String zum Übersetzen"=w212:string)  [unwired: 9 in, 4 out]
            n164 = One Button Dialog(message=w212, button name ("OK")="OK" ("Schaltflächentext (\"OK\")")) -> ()  [unwired: 1 out]
          }
        }
      }
      event "Abbrechen": Value Change {
        n165 = event-data() -> ()  [unwired: 1 in, 6 out]
        n166 = call "Test Status.vi"("Aktion"=Aktion_Test_Status."lesen") -> ("Aktive Tests"=w220:T30, "Tests sperren"=w218:bool)  [unwired: 11 in, 2 out]
        n167 = Unbundle By Name(w220) -> ("ANR läuft"=w219:bool)
        n168 = And(x=w219, y=w218) -> (x .and. y?=w217:bool)
        n169 = case shown="True" w217 {
          tunnel: [w223 w224] -> w222
          tunnel: w216 -> [w223 _]
          frame False {
          }
          frame True {
            n170 = call "FGV-Funktionstasten.vi"("Herkunft"="ANR Test", "Zustand"=Zustaende."Standby", "Aktion"=Funktionstasten-Aktion."Zustand setzen") -> ()  [unwired: 5 in, 8 out]
            n171 = call "FGV ARN Test.vi"("abgebrochen"=TRUE, "Aktion"=Aktion_FGV_ARN_Test."fertig") -> ("Aktion"=w224:T13)  [unwired: 6 in, 3 out]
          }
        }
      }
      event "Textfile": Value Change {
        n172 = event-data() -> ()  [unwired: 1 in, 6 out]
        n173 = call "FGV ARN Protokoll.vi"("Aktion"=Aktion_FGV_ARN_Protokoll."Textdatei speichern") -> ()  [unwired: 8 in, 3 out]
      }
    }
  }
